vi "str to datetimearray.vi"(2 "String":string) -> (6 "timestamp array":timestamp[](array[timestamp]))   [LabVIEW 2013, in "CreateOPCUAServerAuto.lvlib"]
uses:
  CreateOPCUAServerAuto.lvlib
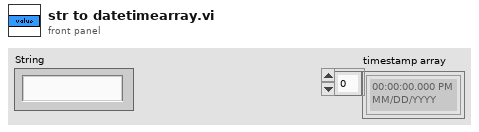
[diagram p1: front panel]
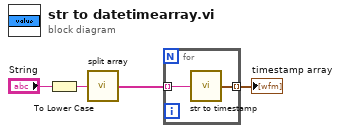
[diagram p0: block diagram]
diagram:
  n1 = To Lower Case(string="String") -> (all lower case string=w3:string)
  n2 = call "split array.vi"("string"=w3) -> ("split arr"=w2:string[])  [unwired: 8 in]
  n3 = for {
    tunnel: w2 -> [w6] mode=indexing
    tunnel: [w5] -> w1 mode=indexing
    n4 = call "str to timestamp.vi"("date/time string"=w6) -> ("Resulting Time Stamp"=w5:timestamp)
  }
  "timestamp array" <- w1
